vi "LOC subReadWriteVIStringINIKeys(String).vi"(4 "Mode":enum16{"Read", "Write"}(ring), 5 "Section":string, 6 "error in (no error)":errorcluster, 8 "ConfigFileRefnum":T1, 9 "ControlRefnum":refnum<vi>) -> (0 "error out":errorcluster)   [LabVIEW 2020, in "Localization_Tools.lvlib"]
uses:
  Localization_Tools.lvlib
  <vilib>/Utility/config.llb/Config Data RefNum.ctl
  <vilib>/Utility/config.llb/NI_LVConfig.lvlib
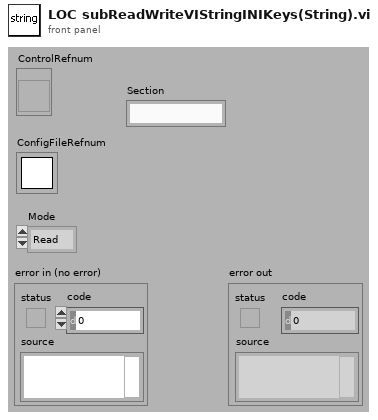
[diagram p1: front panel]
types:
  T1 = typedef "NI_LVConfig.lvlib/Config Data RefNum.ctl" = refnum<k1>
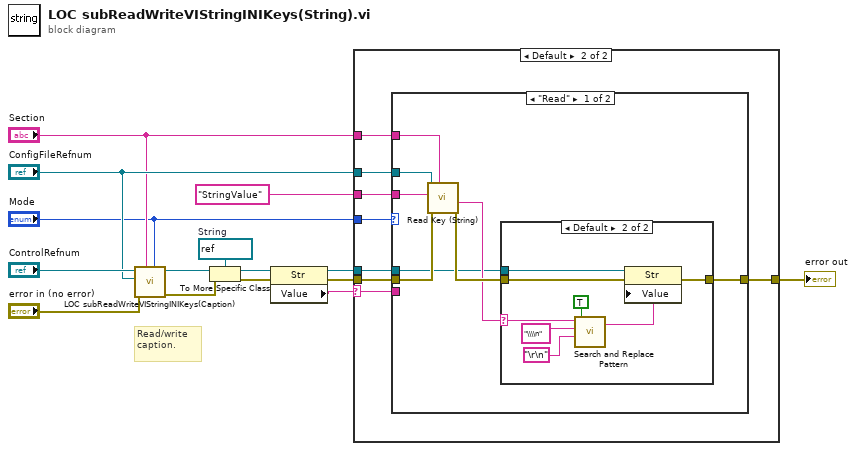
[diagram p0: block diagram]
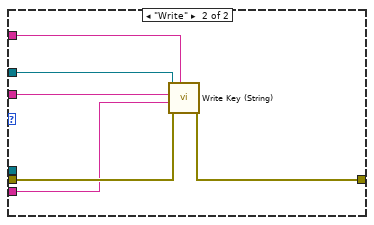
[diagram p4: hidden frame]
diagram:
  w8 = refnum<vi> refnum  # String
  # "Read/write\ncaption."
  n1 = call "LOC subReadWriteVIStringINIKeys(Caption).vi"("Mode"="Mode", "Section"="Section", "error in (no error)"="error in (no error)", "ConfigFileRefnum"="ConfigFileRefnum", "ControlRefnum"="ControlRefnum") -> ("error out"=w6:errorcluster, "dup ControlRefnum"=w7:refnum<vi>)  [unwired: 3 in]
  n2 = To More Specific Class(target class=w8, reference=w7, error in=w6) -> (specific class reference=w5:refnum<vi>, error out=w4:errorcluster)
  n3 = property class="Str"(reference=w5, error in=w4) -> (reference out=w2:refnum<vi>, error out=w3:errorcluster, "Value"=w1:string)
  n4 = case shown="Default" w1 {
    selector: w1 -> [_ w17]
    tunnel: "StringValue" ("key") -> [_ w24]
    tunnel: "ConfigFileRefnum" -> [_ w23]
    tunnel: "Section" -> [_ w22]
    tunnel: "Mode" -> [_ w21]
    tunnel: [w16 w20] -> w9
    tunnel: w3 -> [w16 w19]
    tunnel: w2 -> [_ w18]
    frame "" {
    }
    frame Default {
      n5 = case shown="\"Read\"" w21 {
        tunnel: w18 -> [w25 _]
        tunnel: w19 -> [w26 w43]
        tunnel: w23 -> [w32 w47]
        tunnel: w22 -> [w31 w45]
        tunnel: w24 -> [w30 w46]
        tunnel: [w28 w44] -> w20
        tunnel: w17 -> [_ w42]
        frame "Read" {
          n6 = call <vilib>:"Read Key (String).vi"("section"=w31, "error in (no error)"=w26, "key"=w30, "refnum"=w32) -> ("error out"=w29:errorcluster, "value"=w27:string)  [unwired: 4 in, 2 out]
          n7 = case shown="Default" w27 {
            selector: w27 -> [_ w38]
            tunnel: w25 -> [_ w41]
            tunnel: w29 -> [w33 w40]
            tunnel: [w33 w39] -> w28
            frame "" {
            }
            frame Default {
              n8 = call <vilib>:"Search and Replace Pattern.vi"("string"=w38, "regular expression (\"\")"="\\\\n" ("regular expression (\"\")"), "replace string (\"\")"="\r\n", "replace all? (F)"=TRUE) -> ("result string"=w34:string)  [unwired: 1 in, 1 out]
              n9 = property class="Str"(reference=w41, error in=w40, "Value"=w34) -> (error out=w39:errorcluster)  [unwired: 1 out]
            }
          }
        }
        frame "Write" {
          n10 = call <vilib>:"Write Key (String).vi"("section"=w45, "error in (no error)"=w43, "value"=w42, "key"=w46, "refnum"=w47) -> ("error out"=w44:errorcluster)  [unwired: 4 in, 2 out]
        }
      }
    }
  }
  "error out" <- w9
